vi "MissionControl2017 - MAIN.vi"() -> ()   [LabVIEW 2015, in "MissionControl2017.lvlib"]
uses:
  MissionControl2017.lvlib
  PathfindingSettings.ctl
  MovementSettings.ctl
  PathCostWeights.ctl
  IntermediatePositionGrids.ctl
  <vilib>/Utility/miscctls.llb/LVPoint32TypeDef.ctl
  LocalizationStatus.ctl
  <vilib>/Utility/miscctls.llb/LVBoundsTypeDef.ctl
  Vector.ctl
  PathOfMoves.ctl
  Move.ctl
  Overlord2017.lvlib
  SubVIs - MissionControl2017.lvlib
  TestbenchUtils - Navigation2017.lvlib
  Types - Navigation2017.lvlib
  <vilib>/sound2/lvsound2.llb/Sampling Mode.ctl
  <vilib>/sound2/lvsound2.llb/Sound Data Format.ctl
  <vilib>/sound2/lvsound2.llb/Sound File Position.ctl
  <vilib>/sound2/lvsound2.llb/Sound Output Write (DBL).vi
panel:
  out "appended path":path
  in  "WaitingForLocalization":bool=TRUE
  in  "Timer Reset":bool
  out "Timer (ms)":u32=89862
  in  "Movement Control Turn Tightness":dbl(slide)=6.226706181197886 scale=1.0..10.0
  out "Right Motor PWM":dbl(graph)
  out "Left Motor PWM":dbl(graph)
  out "Motor PWM XY Graph":cluster{"X":dbl, "Y":dbl}[](graph)
  out "Position at Start of Pathfinding Calculation":T1={"x"=0.8634599999999999, "y"=2.6651953125, "angle"=-0.39269908169872414, "valid"=TRUE, "lastUpdatedTime"=858996870.0}
  out "Current Localization Status (As Drawn Above)":T1={"x"=2.07378, "y"=1.550390625, "angle"=-1.9634954084936207, "valid"=TRUE, "lastUpdatedTime"=859077686.0}
  in  "Debug Mining":bool=TRUE
  in  "Debug Wheel Motors":bool=TRUE
  out "navDebugBotSpin":dbl=-1.9634954084936207
  out "y (m)":dbl=0.3912890625
  out "x (m)":dbl=5.97042
  in  "Debug Localization - Mouse":bool=TRUE
  out "Mouse Wheel Sum":dbl=1.0
  out "Mouse Wheel Delta":i32=1
  out "Mouse Down Button":u16=1
  out "Mouse Coords":T2={"Horizontal"=191, "Vertical"=53}
  out "Mouse Down Coords":T2={"Horizontal"=719, "Vertical"=210}
  out "CurrMiningRun":i16(slide) scale=0.0..3.0
  out "CurrStage":string="Spinning & Moving to Mining Area"
  out "UsedDesperation":bool
  out "SpecifyingEndAngle":bool=TRUE
  out "NextPointIsDestination":bool
  out "CurrNavStage":string="Stopping robot (brief pause)"
  out "FPS Indicator":bool=TRUE
  in  "Pathfinding Settings":T3={"Movement Settings"={"Arrival Tolerance (m)"=0.01, "Closeness Threshold (m)"=0.5, "Pit Obstacle Radius (m)"=0.5, "Pit Locations"=[]}, "Dead Zone"=0.75, "Max Moves"=2.0, "Move Segment Length (m)"=0.2, "Path Cost Weights"={"Length Weight"=1.0, "Angle Weight"=0.0, "Angle Error Weight"=1000.0, "Angle Error Threshold"=0.314, "Per Move Penalty"=0.05, "Closeness Weight"=100.0, "Too Short Penalty"=100.0, "Too Short Threshold"=1.5}, "Desperation - Reduction Per Attempt (Ratio)"=0.9, "Desperation - Max Attempts"=1, "Log All Move Points"=TRUE, "Intermediate Position Grids"=[{"x1"=0.0, "x2"=1.75, "resolution"=0.15}, {"x1"=1.75, "x2"=7.38, "resolution"=0.4}]}
  out "Arena Pixel Size":i16[](array[numeric])=[1000, 512]
  out "Arena Control":picture
  # "NOTE: Open and pin\n\nMineOrDumpBlocking.vi\nand\nSetWheelMotorPWM.vi\n\nalongside when debugging."
  # "(Spin robot with arrow keys)"
  # "To toggle localization debugging:\n- Flip this switch <---\n- Set the Project Property -> Conditional Compilation Property\n\"DISCONNECT_LOCALIZATION\" to True or False"
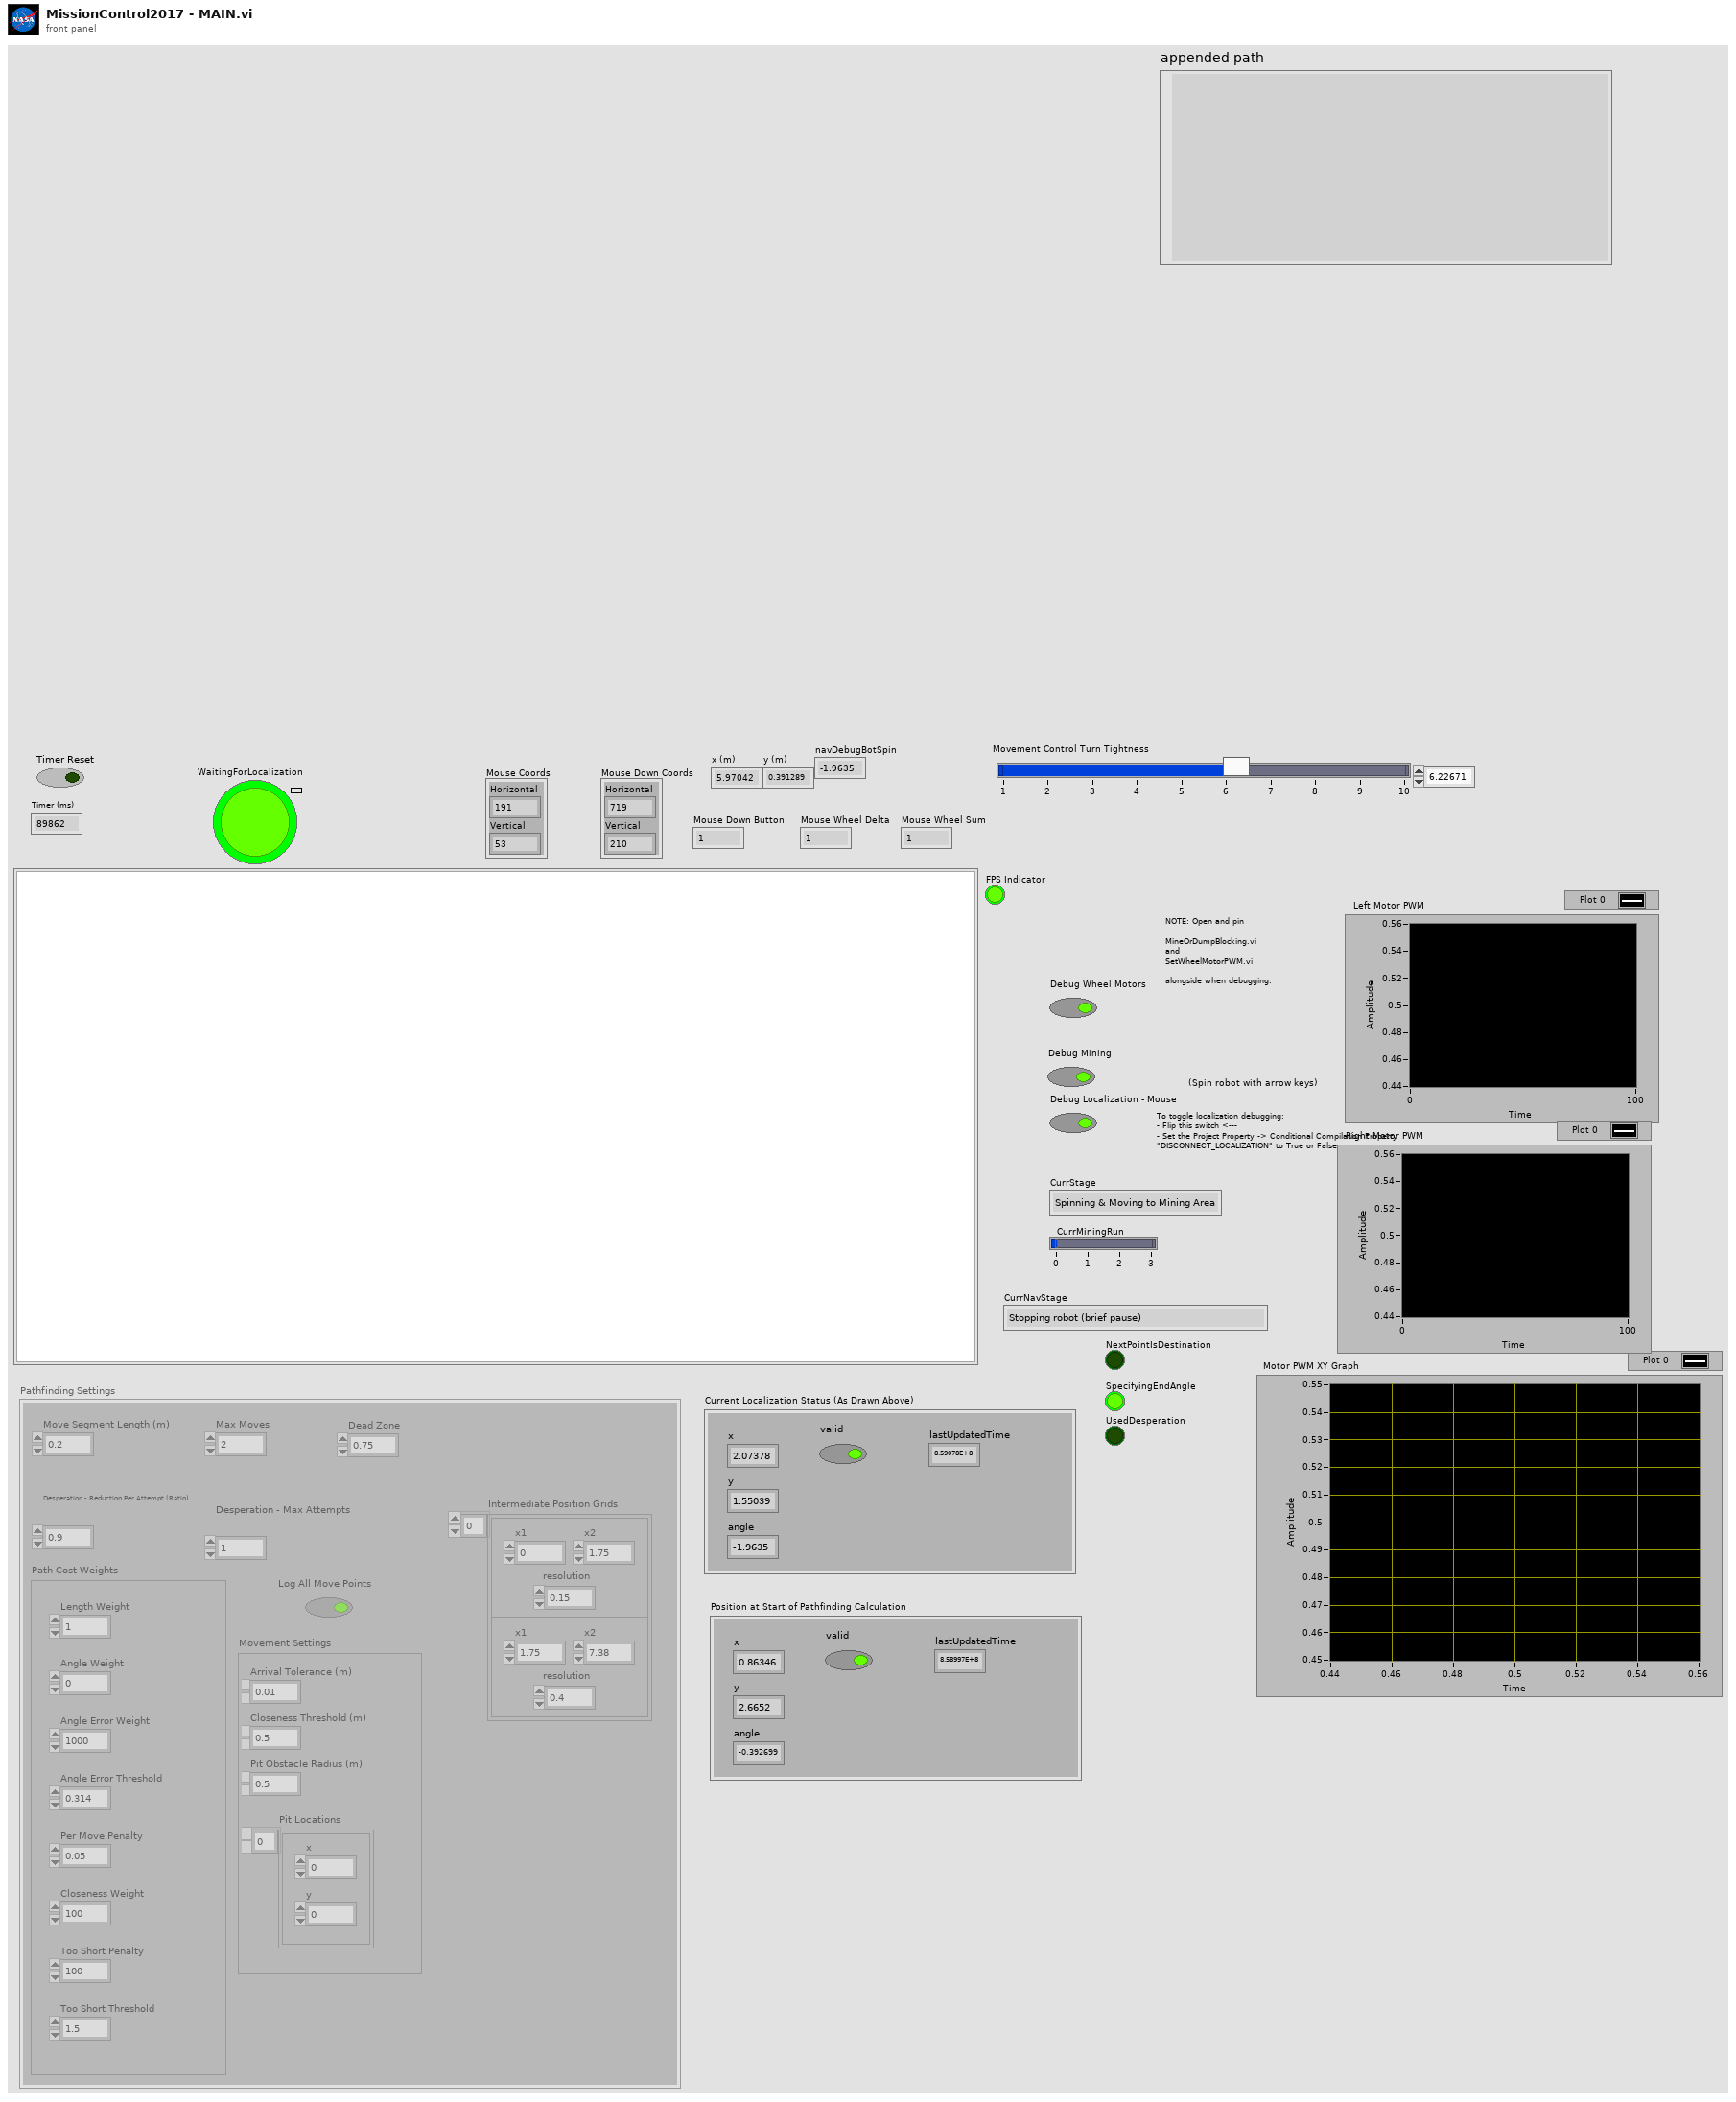
[diagram p1: front panel]
types:
  T1 = typedef "Navigation2017.lvlib/TestbenchUtils - Navigation2017.lvlib/LocalizationStatus.ctl" = cluster{"x":dbl, "y":dbl, "angle":dbl, "valid":bool, "lastUpdatedTime":dbl}
  T2 = typedef "LVPoint32TypeDef.ctl" = cluster{"Horizontal":i32, "Vertical":i32}
  T3 = typedef "Navigation2017.lvlib/Types - Navigation2017.lvlib/PathfindingSettings.ctl" = cluster{"Movement Settings":T4, "Dead Zone":dbl, "Max Moves":dbl, "Move Segment Length (m)":dbl, "Path Cost Weights":T5, "Desperation - Reduction Per Attempt (Ratio)":dbl, "Desperation - Max Attempts":i16, "Log All Move Points":bool, "Intermediate Position Grids":T6}
  T4 = typedef "Navigation2017.lvlib/Types - Navigation2017.lvlib/MovementSettings.ctl" = cluster{"Arrival Tolerance (m)":dbl, "Closeness Threshold (m)":dbl, "Pit Obstacle Radius (m)":dbl, "Pit Locations":cluster{"x":dbl, "y":dbl}[]}
  T5 = typedef "Navigation2017.lvlib/Types - Navigation2017.lvlib/PathCostWeights.ctl" = cluster{"Length Weight":dbl, "Angle Weight":dbl, "Angle Error Weight":dbl, "Angle Error Threshold":dbl, "Per Move Penalty":dbl, "Closeness Weight":dbl, "Too Short Penalty":dbl, "Too Short Threshold":dbl}
  T6 = typedef "Navigation2017.lvlib/Types - Navigation2017.lvlib/IntermediatePositionGrids.ctl" = cluster{"x1":dbl, "x2":dbl, "resolution":dbl}[]
  T7 = typedef "LVBoundsTypeDef.ctl" = cluster{"Width":u32, "Height":u32}
  T8 = typedef "eventvkey.ctl" = enum16{"ASCII", "Enter", "Return", "Shift", "Ctrl", "Alt", "Cmd", "Opt", "Caps", "NumLock", "Clear", "Break", "Up", "Down", "Left", "Right", "Insert", "Delete", "Home", "End", "PageUp", "PageDown", "Escape", "Help", "Pause", "ScrollLock", "F1", "F2", "F3", "F4", "F5", "F6", "F7", "F8", "F9", "F10", "F11", "F12", "F13", "F14", "F15", "F16", "F17", "F18", "F19", "F20", "F21", "F22", "F23", "F24", "Play", "VolumeUp", "VolumeDown", "Mute", "Two Byte Char"}
  T9 = typedef "imagedata.ctl" = cluster{"image type":i32, "image depth":i32, "image":u8[], "mask":u8[], "colors":u32[], "Rectangle":cluster{"left":i16, "top":i16, "right":i16, "bottom":i16}}
  T10 = cluster{"Width":u16, "Style":enum32{"Solid", "Dash", "Dot", "DashDot", "DashDotDot"}}
  T11 = typedef "Navigation2017.lvlib/Types - Navigation2017.lvlib/Vector.ctl" = cluster{"x":dbl, "y":dbl, "angle":dbl}
  T12 = typedef "Navigation2017.lvlib/Types - Navigation2017.lvlib/PathOfMoves.ctl" = cluster{"Dest Angle Error":dbl, "Dest Angle Considered":bool, "Moves":T13[]}
  T13 = typedef "Navigation2017.lvlib/Types - Navigation2017.lvlib/Move.ctl" = cluster{"Did Reach Dest":bool, "Did Collide":bool, "Sum of Angle Changes (rad)":dbl, "Move Length (m)":dbl, "Closeness Sum":dbl, "Positions Along Move":T11[], "Moved Fwd":bool}
  T14 = typedef "Sound Data Format.ctl" = cluster{"sample rate (S/s)":dbl, "number of channels":i32, "bits per sample":i32}
  T15 = typedef "Sampling Mode.ctl" = i32
  T16 = typedef "Sound Output Task ID.ctl" = u32
  T17 = typedef "Sound File Position.ctl" = u16
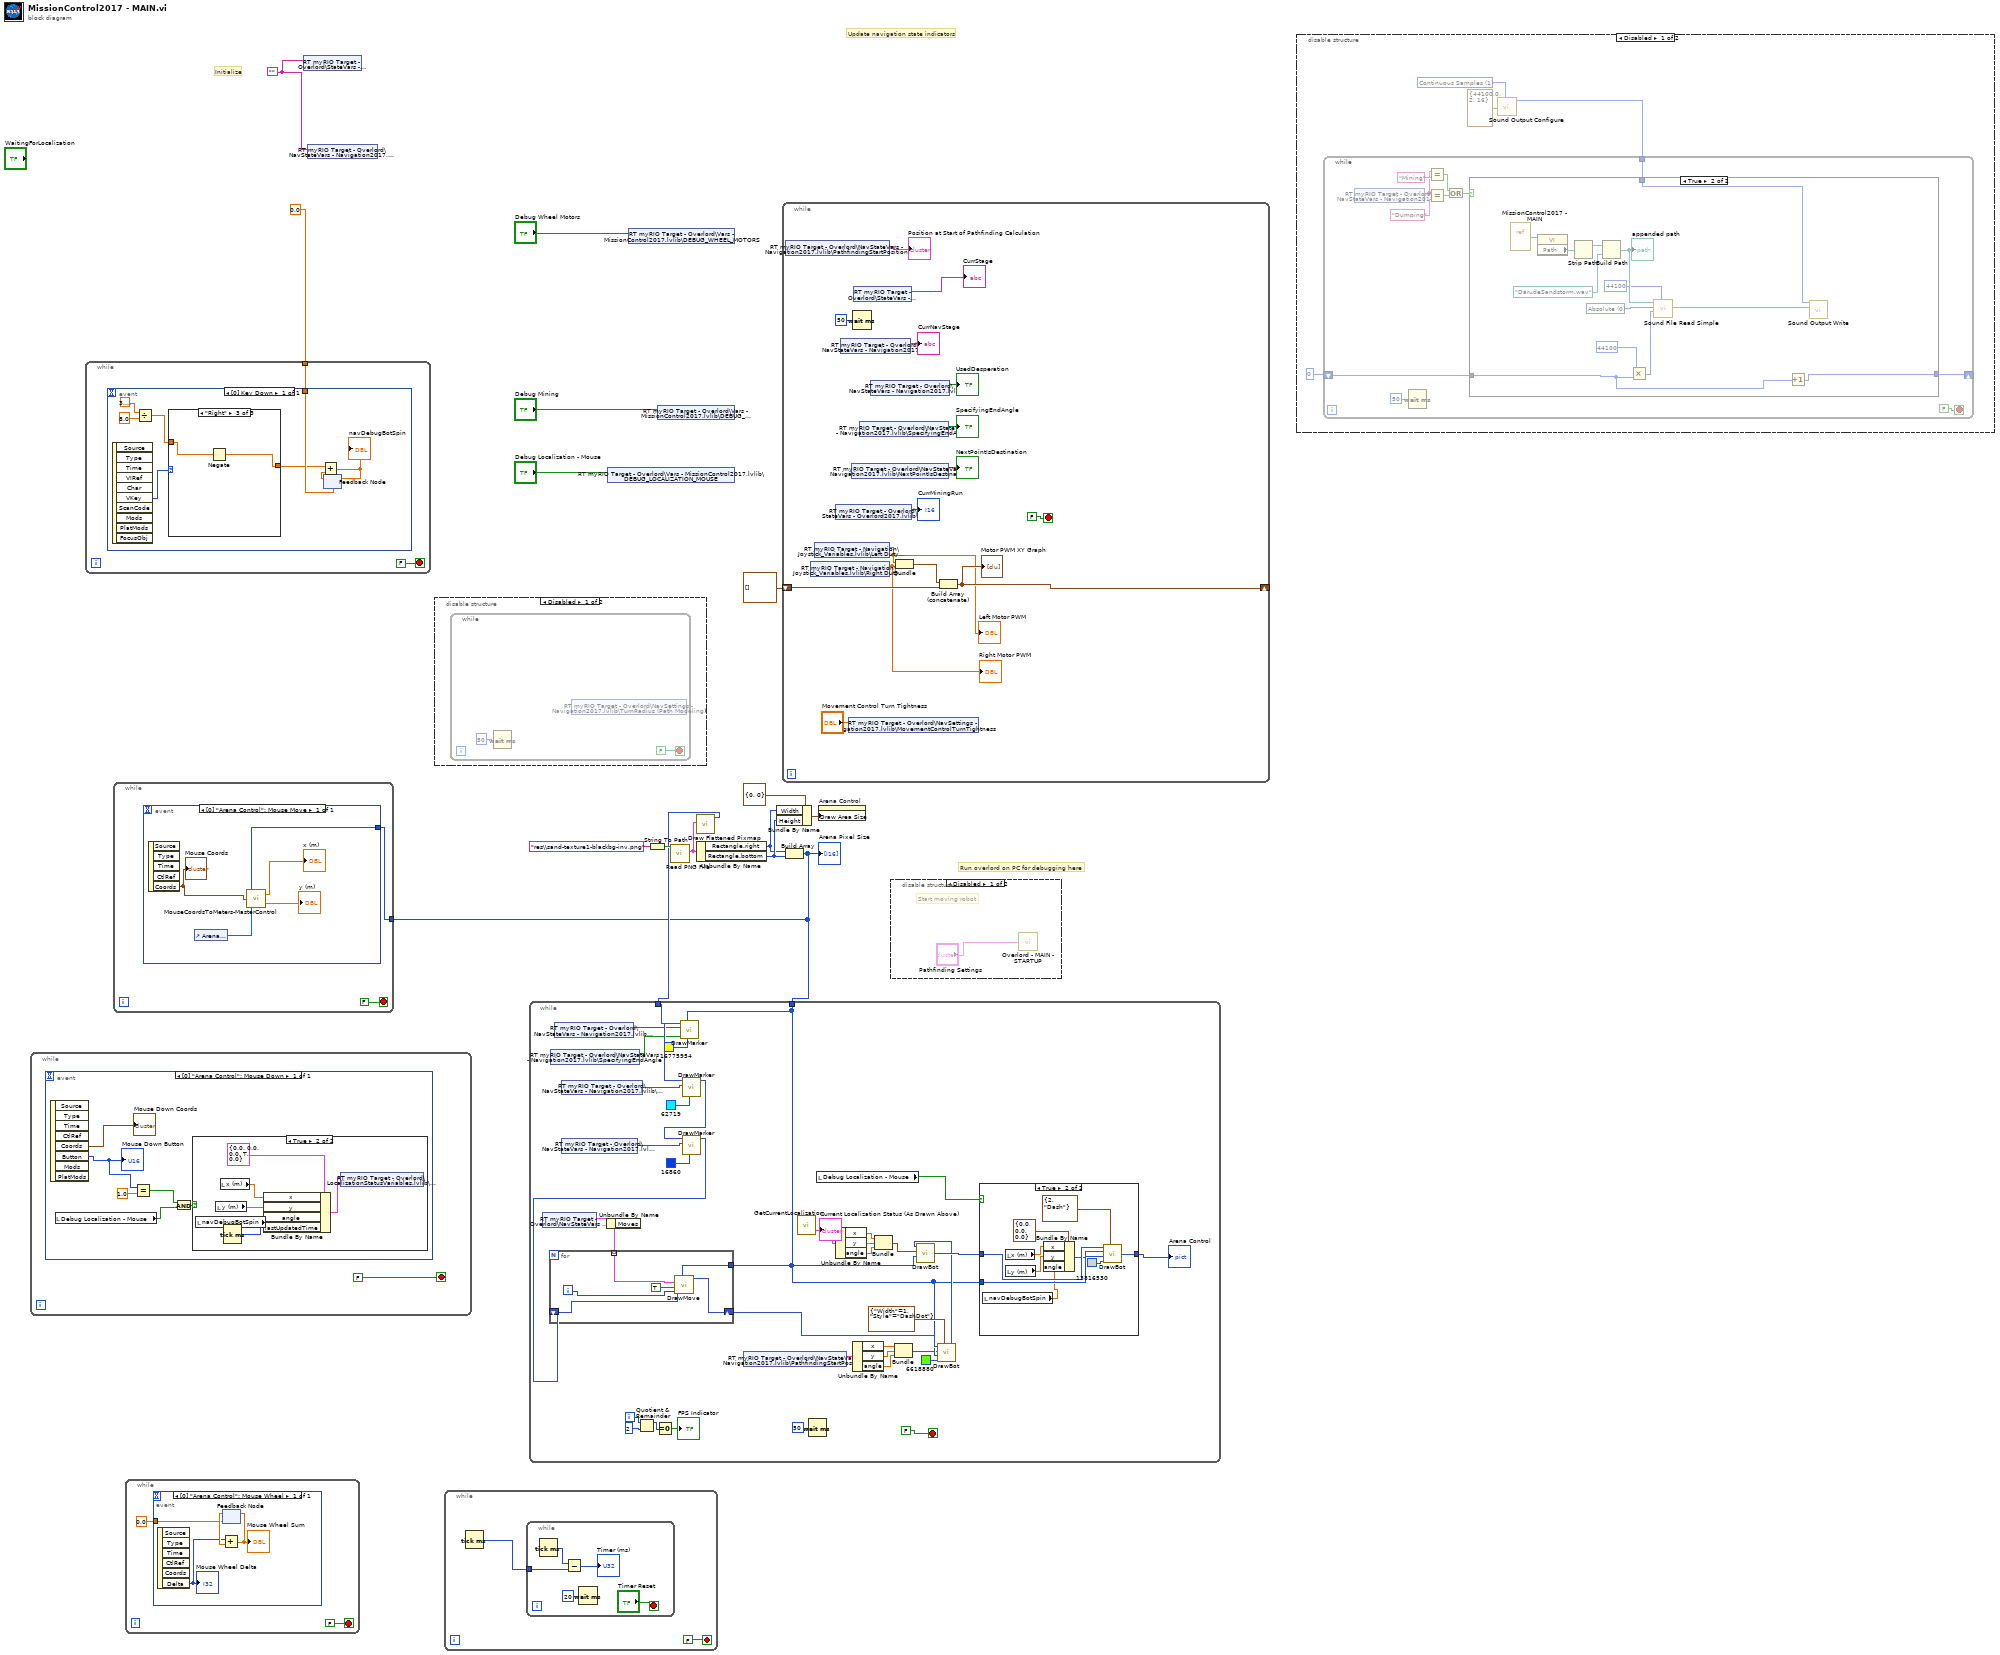
[diagram p0: block diagram]
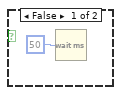
[diagram p3: hidden frame]
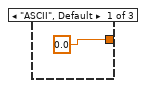
[diagram p6: hidden frame]
diagram:
  w5 = ""
  # "Run overlord on PC for debugging here"
  # "Initialize"
  # "Update navigation state indicators"
  n1 = while {
    stop <- FALSE stop-if-true
    n2 = event shown="[0] \"Arena Control\": Mouse Down" {
      selector: _ -> [_]
      dyn-events: _ -> [_]
      timeout: _ -> [_]
      event "Arena Control": Mouse Down {
        n3 = event-data() -> ("Coords"=→"Mouse Down Coords":T2, "Button"=w20:u16)  [unwired: 1 in, 6 out]
        "Mouse Down Button" <- w20
        n4 = local read "Debug Localization - Mouse"() -> (w19:bool)
        n5 = Equal?(x=w20, y=1.0) -> (x = y?=w18:bool)
        n6 = And(x=w18, y=w19) -> (x .and. y?=w17:bool)
        n7 = case shown="True" w17 {
          frame False {
          }
          frame True {
            n8 = local read "navDebugBotSpin"() -> (w23:dbl)
            n9 = local read "y (m)"() -> (w24:dbl)
            n10 = local read "x (m)"() -> (w25:dbl)
            n11 = Tick Count (ms)() -> (millisecond timer value=w26:u32)
            n12 = Bundle By Name(cluster=T1 {"x"=0.0, "y"=0.0, "angle"=0.0, "valid"=TRUE, "lastUpdatedTime"=0.0} ("Localization Status"), "x"=w25, "y"=w24, "angle"=w23, "lastUpdatedTime"=w26) -> (w27:T1)
            n13 = shared-variable "RT myRIO Target - Overlord\\LocalizationStatusVariables.lvlib\\LocalizationStatus"(w27) -> ()  [unwired: 1 in, 1 out]
          }
        }
      }
    }
  }
  n14 = while {
    tunnel: 0.0 -> [w29]
    stop <- FALSE stop-if-true
    n15 = event shown="[0] Key Down" {
      selector: _ -> [_]
      dyn-events: _ -> [_]
      timeout: _ -> [_]
      tunnel: w29 -> [w35]
      event Key Down {
        n16 = event-data() -> ("VKey"=w38:T8)  [unwired: 1 in, 9 out]
        n17 = Divide(x=3.141592653589793, y=8.0) -> (x/y=w31:dbl)
        n18 = case shown="\"Right\"" w38 {
          tunnel: [0.0 w40 w41] -> w34
          tunnel: w31 -> [_ w40 w42]
          frame "ASCII", Default {
          }
          frame "Left" {
          }
          frame "Right" {
            n19 = Negate(x=w42) -> (-x=w41:dbl)
          }
        }
        n20 = feedback #1(w35) -> (w36:dbl)
        n21 = Add(x=w34, y=w36) -> (x+y=w37:dbl)
        "navDebugBotSpin" <- w37
        n22 = feedback-in #1(w37) -> ()
      }
    }
  }
  n23 = while {
    stop <- FALSE stop-if-true
    n24 = event shown="[0] \"Arena Control\": Mouse Wheel" {
      selector: _ -> [_]
      dyn-events: _ -> [_]
      timeout: _ -> [_]
      tunnel: 0.0 -> [w46]
      event "Arena Control": Mouse Wheel {
        n25 = event-data() -> ("Delta"=w45:i32)  [unwired: 1 in, 5 out]
        "Mouse Wheel Delta" <- w45
        n26 = feedback #2(w46) -> (w47:dbl)
        n27 = Add(x=w45, y=w47) -> (x+y=w48:dbl)
        "Mouse Wheel Sum" <- w48
        n28 = feedback-in #2(w48) -> ()
      }
    }
  }
  n29 = shared-variable "RT myRIO Target - Overlord\\StateVars - Overlord2017.lvlib\\CurrStage"(w5) -> ()  [unwired: 1 in, 1 out]
  n30 = shared-variable "RT myRIO Target - Overlord\\NavStateVars - Navigation2017.lvlib\\CurrNavStage"(w5) -> ()  [unwired: 1 in, 1 out]
  n31 = disable-structure shown="Disabled" {
    frame Disabled {
      n32 = while {
        stop <- FALSE stop-if-true
        n33 = Wait (ms)(milliseconds to wait=u32 50) -> ()  [unwired: 1 out]
        n34 = shared-variable "RT myRIO Target - Overlord\\NavSettings - Navigation2017.lvlib\\TurnRadius (Path Modeling)"() -> (w51:dbl)  [unwired: 1 in, 1 out]
      }
    }
    frame Enabled {
    }
  }
  n35 = while {
    stop <- FALSE stop-if-true
    n36 = Tick Count (ms)() -> (millisecond timer value=w53:u32)
    n37 = while {
      tunnel: w53 -> [w55]
      stop <- "Timer Reset" stop-if-true
      n38 = Tick Count (ms)() -> (millisecond timer value=w56:u32)
      n39 = Subtract(x=w56, y=w55) -> (x-y=→"Timer (ms)":u32)
      n40 = Wait (ms)(milliseconds to wait=u32 20) -> ()  [unwired: 1 out]
    }
  }
  n41 = shared-variable "RT myRIO Target - Overlord\\Vars - MissionControl2017.lvlib\\DEBUG_LOCALIZATION_MOUSE"("Debug Localization - Mouse") -> ()  [unwired: 1 in, 1 out]
  n42 = shared-variable "RT myRIO Target - Overlord\\Vars - MissionControl2017.lvlib\\DEBUG_WHEEL_MOTORS"("Debug Wheel Motors") -> ()  [unwired: 1 in, 1 out]
  n43 = String To Path(string="res\\sand-texture1-blackbg-inv.png" ("name or relative path")) -> (path=w14:path)
  n44 = shared-variable "RT myRIO Target - Overlord\\Vars - MissionControl2017.lvlib\\DEBUG_BUCKET"("Debug Mining") -> ()  [unwired: 1 in, 1 out]
  n45 = call <vilib>:"Read PNG File.vi"("path to PNG file"=w14) -> ("image data"=w9:T9)  [unwired: 8 in, 2 out]
  n46 = call <vilib>:"Draw Flattened Pixmap.vi"("image data"=w9) -> ("new picture"=w8:picture)  [unwired: 8 in]
  n47 = Unbundle By Name(w9) -> ("Rectangle.right"=w11:i16, "Rectangle.bottom"=w12:i16)
  n48 = Bundle By Name(cluster=T7 {"Width"=0, "Height"=0} ("Draw Area Size"), "Width"=w11, "Height"=w12) -> (w13:T7)
  n49 = while {
    shift-right: [w63] -> _
    shift-left: cluster{"Double":dbl, "Double":dbl}[] [] -> [w64]
    stop <- FALSE stop-if-true
    n50 = shared-variable "RT myRIO Target - Overlord\\NavStateVars - Navigation2017.lvlib\\PathfindingStartPosition"() -> (→"Position at Start of Pathfinding Calculation":T1)  [unwired: 1 in, 1 out]
    n51 = shared-variable "RT myRIO Target - Navigation\\Joystick_Variables.lvlib\\Right Duty Cycle"() -> (w62:dbl)  [unwired: 1 in, 1 out]
    "Right Motor PWM" <- w62
    n52 = shared-variable "RT myRIO Target - Navigation\\Joystick_Variables.lvlib\\Left Duty Cycle"() -> (w61:dbl)  [unwired: 1 in, 1 out]
    "Left Motor PWM" <- w61
    n53 = shared-variable "RT myRIO Target - Overlord\\StateVars - Overlord2017.lvlib\\CurrMiningRun"() -> (→"CurrMiningRun":i16)  [unwired: 1 in, 1 out]
    n54 = shared-variable "RT myRIO Target - Overlord\\NavStateVars - Navigation2017.lvlib\\CurrNavStage"() -> (→"CurrNavStage":string)  [unwired: 1 in, 1 out]
    n55 = shared-variable "RT myRIO Target - Overlord\\NavSettings - Navigation2017.lvlib\\MovementControlTurnTightness"("Movement Control Turn Tightness") -> ()  [unwired: 1 in, 1 out]
    n56 = shared-variable "RT myRIO Target - Overlord\\NavStateVars - Navigation2017.lvlib\\NextPointIsDestination"() -> (→"NextPointIsDestination":bool)  [unwired: 1 in, 1 out]
    n57 = Wait (ms)(milliseconds to wait=u32 50) -> ()  [unwired: 1 out]
    n58 = shared-variable "RT myRIO Target - Overlord\\StateVars - Overlord2017.lvlib\\CurrStage"() -> (→"CurrStage":string)  [unwired: 1 in, 1 out]
    n59 = shared-variable "RT myRIO Target - Overlord\\NavStateVars - Navigation2017.lvlib\\SpecifyingEndAngle"() -> (→"SpecifyingEndAngle":bool)  [unwired: 1 in, 1 out]
    n60 = shared-variable "RT myRIO Target - Overlord\\NavStateVars - Navigation2017.lvlib\\UsedDesperation"() -> (→"UsedDesperation":bool)  [unwired: 1 in, 1 out]
    n61 = Bundle("Double"=w61, "Double"=w62) -> (w65:cluster{"Double":dbl, "Double":dbl})  [unwired: 1 in]
    n62 = Build Array (concatenate)(w65, w64) -> (w63:cluster{"Double":dbl, "Double":dbl}[])
    "Motor PWM XY Graph" <- w63
  }
  n63 = Build Array(w11, w12) -> (w6:i16[])
  "Arena Pixel Size" <- w6
  n64 = while {
    tunnel: w6 -> [w74]
    stop <- FALSE stop-if-true
    n65 = event shown="[0] \"Arena Control\": Mouse Move" {
      selector: _ -> [_]
      dyn-events: _ -> [_]
      timeout: _ -> [_]
      tunnel: w74 -> [w79]
      event "Arena Control": Mouse Move {
        n66 = event-data() -> ("Coords"=w80:T2)  [unwired: 1 in, 4 out]
        "Mouse Coords" <- w80
        n67 = control-ref of="Arena Control"() -> (w78:refnum<vi>)
        n68 = call "MouseCoordsToMeters-MasterControl.vi"("Picture Control Ref"=w78, "Mouse Pos"=w80, "Arena Pixel Dim"=w79) -> ("y (m)"=→"y (m)":dbl, "x (m)"=→"x (m)":dbl)
      }
    }
  }
  n69 = while {
    tunnel: w8 -> [w101]
    tunnel: w6 -> [w90]
    i -> [w116]
    stop <- FALSE stop-if-true
    n70 = shared-variable "RT myRIO Target - Overlord\\NavStateVars - Navigation2017.lvlib\\CurrPath"() -> (w104:T12)  [unwired: 1 in, 1 out]
    n71 = shared-variable "RT myRIO Target - Overlord\\NavStateVars - Navigation2017.lvlib\\SpecifyingEndAngle"() -> (w95:bool)  [unwired: 1 in, 1 out]
    n72 = shared-variable "RT myRIO Target - Overlord\\NavStateVars - Navigation2017.lvlib\\DestinationPoint"() -> (w96:T11)  [unwired: 1 in, 1 out]
    n73 = shared-variable "RT myRIO Target - Overlord\\NavStateVars - Navigation2017.lvlib\\NextPointOnPath"() -> (w97:T11)  [unwired: 1 in, 1 out]
    n74 = shared-variable "RT myRIO Target - Overlord\\NavStateVars - Navigation2017.lvlib\\CurrPosOnPath"() -> (w84:T11)  [unwired: 1 in, 1 out]
    n75 = Unbundle By Name(w104) -> ("Moves"=w103:T13[])
    n76 = Quotient & Remainder(x=w116, y=2) -> (x-y*floor(x/y)=w107:i32)  [unwired: 1 out]
    n77 = Equal To 0?(x=w107) -> (x = 0?=→"FPS Indicator":bool)
    n78 = call "DrawMarker.vi"("color(black)"=u32 16775954, "Arena Pixel Dim"=w90, "Draw An Arrow"=w95, "Cluster"=w96, "picture in"=w101) -> ("new picture"=w102:picture)  [unwired: 6 in]
    n79 = call "DrawMarker.vi"("color(black)"=u32 62719, "Cluster"=w97, "picture in"=w102) -> ("new picture"=w82:picture)  [unwired: 8 in]
    n80 = call "DrawMarker.vi"("color(black)"=u32 16860, "Cluster"=w84, "picture in"=w82) -> ("new picture"=w81:picture)  [unwired: 8 in]
    n81 = for {
      tunnel: w90 -> [w121]
      shift-right: [w122] -> w94
      shift-left: w81 -> [w123]
      tunnel: w103 -> [w119] mode=indexing
      i -> [w118]
      n82 = call "DrawMove.vi"("Arena Pixel Dim"=w121, "Move Number (optional)"=w118, "Show Vectors?"=TRUE, "Move"=w119, "picture in"=w123) -> ("picture out"=w122:picture)  [unwired: 3 in]
    }
    n83 = shared-variable "RT myRIO Target - Overlord\\NavStateVars - Navigation2017.lvlib\\PathfindingStartPosition"() -> (w88:T1)  [unwired: 1 in, 1 out]
    n84 = call "GetCurrentLocalization.vi"() -> ("Current Localization Status"=w109:T1)  [unwired: 1 out]
    "Current Localization Status (As Drawn Above)" <- w109
    n85 = Wait (ms)(milliseconds to wait=u32 50) -> ()  [unwired: 1 out]
    n86 = local read "Debug Localization - Mouse"() -> (w98:bool)
    n87 = Unbundle By Name(w109) -> ("x"=w112:dbl, "y"=w111:dbl, "angle"=w110:dbl)
    n88 = Unbundle By Name(w88) -> ("x"=w87:dbl, "y"=w86:dbl, "angle"=w85:dbl)
    n89 = Bundle("x"=w112, "y"=w111, "angle"=w110) -> (w108:cluster{"x":dbl, "y":dbl, "angle":dbl})  [unwired: 1 in]
    n90 = Bundle("x"=w87, "y"=w86, "angle"=w85) -> (w89:cluster{"x":dbl, "y":dbl, "angle":dbl})  [unwired: 1 in]
    n91 = call "DrawBot.vi"("picture in"=w94, "bot pos vector"=w89, "Arena Pixel Size"=w90, "bot color"=u32 6618880, "pen"=T10 {"Width"=1, "Style"=enum."DashDot"}) -> ("picture out"=w93:picture)
    n92 = call "DrawBot.vi"("picture in"=w93, "bot pos vector"=w108, "Arena Pixel Size"=w90) -> ("picture out"=w106:picture)  [unwired: 2 in]
    n93 = case shown="True" w98 {
      tunnel: w106 -> [w124 w134]
      tunnel: [w124 w133] -> w105
      tunnel: w90 -> [_ w130]
      frame False {
      }
      frame True {
        n94 = local read "navDebugBotSpin"() -> (w125:dbl)
        n95 = local read "x (m)"() -> (w127:dbl)
        n96 = local read "y (m)"() -> (w128:dbl)
        n97 = Bundle By Name(cluster=T11 {"x"=0.0, "y"=0.0, "angle"=0.0} ("Vector"), "x"=w127, "y"=w128, "angle"=w125) -> (w129:T11)
        n98 = call "DrawBot.vi"("picture in"=w134, "bot pos vector"=w129, "Arena Pixel Size"=w130, "bot color"=u32 13816530, "pen"=T10 {"Width"=2, "Style"=enum."Dash"}) -> ("picture out"=w133:picture)
      }
    }
    "Arena Control" <- w105
  }
  n99 = property on="Arena Control" class="Pict"("Draw Area Size"=w13) -> ()  [unwired: 2 in, 2 out]
  n100 = disable-structure shown="Disabled" {
    frame Disabled {
      # "Start moving robot"
      n101 = call "Overlord - MAIN - STARTUP.vi"("Pathfinding Settings"="Pathfinding Settings") -> ()
    }
    frame Enabled {
    }
  }
  n102 = disable-structure shown="Disabled" {
    frame Disabled {
      w138 = T15 1 items=["Finite Samples", "Continuous Samples"] ("sample mode")
      n103 = call <vilib>:"Sound Output Configure.vi"("sample mode"=w138, "sound format"=T14 {"sample rate (S/s)"=44100.0, "number of channels"=2, "bits per sample"=16}) -> ("task ID"=w137:T16)  [unwired: 8 in, 1 out]
      n104 = while {
        tunnel: w137 -> [w142]
        shift-right: [w141] -> _
        shift-left: 0 -> [w140]
        stop <- FALSE stop-if-true
        n105 = shared-variable "RT myRIO Target - Overlord\\NavStateVars - Navigation2017.lvlib\\CurrNavStage"() -> (w145:string)  [unwired: 1 in, 1 out]
        n106 = Wait (ms)(milliseconds to wait=u32 50) -> ()  [unwired: 1 out]
        n107 = Equal?(x=w145, y="Mining") -> (x = y?=w149:bool)
        n108 = Equal?(x=w145, y="Dumping") -> (x = y?=w148:bool)
        n109 = Or(x=w149, y=w148) -> (x .or. y?=w144:bool)
        n110 = case shown="True" w144 {
          tunnel: w142 -> [_ w155]
          tunnel: [_ w153] -> w141
          tunnel: w140 -> [_ w152]
          frame False {
            n111 = Wait (ms)(milliseconds to wait=u32 50) -> ()  [unwired: 1 out]
          }
          frame True {
            w164 = T17 0 items=["Absolute"=0, "Relative"=2] ("position mode")
            n112 = vi-ref "MissionControl2017 - MAIN.vi"() -> (w160:refnum<vi>)
            n113 = property class="VI"(reference=w160) -> ("Path"=w161:path)  [unwired: 1 in, 2 out]
            n114 = Strip Path(path=w161) -> (stripped path=w162:path)  [unwired: 1 out]
            n115 = Build Path(base path=w162, name or relative path=path "DarudeSandstorm.wav" ("path")) -> (appended path=w159:path)
            "appended path" <- w159
            n116 = Multiply(x=44100 ("position offset"), y=w152) -> (x*y=w154:i32)
            n117 = call <vilib>:"Sound File Read Simple.vi"("number of samples/ch (-1: all)"=44100, "position offset"=w154, "position mode"=w164, "path"=w159) -> ("data"=w156:waveform(dbl)[])  [unwired: 4 in, 3 out]
            n118 = Increment(x=w152) -> (x+1=w153:i32)
            n119 = call-poly <vilib>:"Sound Output Write.vi"("data"=w156, "task ID"=w155) -> ()  [unwired: 8 in, 2 out]
          }
        }
      }
    }
    frame Enabled {
    }
  }
